vi "Protected Write (0D U8).vi"(8 "error in (no error)":errorcluster, 9 "offset (0)":u64 format="%d bytes", 10 "value in":u8, 11 "Pointer in":refnum<class "Pointer.lvclass">) -> (0 "error out":errorcluster, 1 "offset out":u64 format="%d bytes", 2 "value out":u8, 3 "Pointer out":refnum<class "Pointer.lvclass">)   [LabVIEW 2017, in "Memory Manager.lvlib" / "Pointer.lvclass"]
doc: "Writes the provided <b>value</b> to the address specified by <b>pointer + offset</b>.\n\n<b>Note:</b> This VI is <b>safe</b>.\n\nSafe means that this function evaluates the size parameter of <b>pointer</b> to ensure that is inbounds of allocated memory before peforming a memory read/write. Reading/writing more data to a pointer than it has allocated can corrupt or crash LabVIEW."
uses:
  Pointer.lvclass
  Write/Write (0D U8).vi
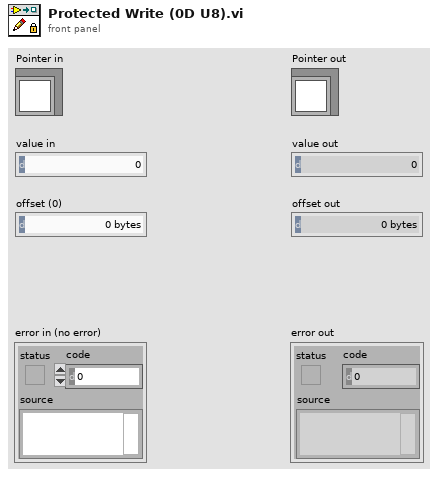
[diagram p1: front panel]
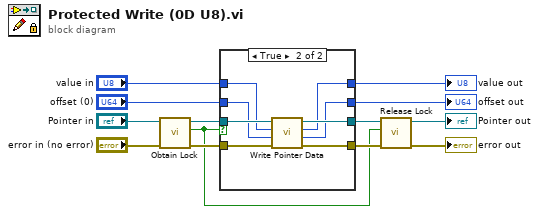
[diagram p0: block diagram]
diagram:
  n1 = call-dynamic "Obtain Lock.vi"("error in (no error)"="error in (no error)", "Pointer in"="Pointer in") -> ("error out"=w11:errorcluster, "lock status"=w9:bool, "Pointer out"=w12:refnum<class "Pointer.lvclass">)  [unwired: 6 in, 1 out]
  n2 = case shown="True" w9 {
    tunnel: [w17 w25] -> w13
    tunnel: [w14 w24] -> w3
    tunnel: [w15 w23] -> w4
    tunnel: w12 -> [w17 w22]
    tunnel: w11 -> [w16 w21]
    tunnel: "value in" -> [w14 w20]
    tunnel: "offset (0)" -> [w15 w19]
    tunnel: [w16 w18] -> w10
    frame False {
    }
    frame True {
      n3 = call-poly "Write Pointer Data.vi"("error in (no error)"=w21, "offset (0)"=w19, "value"=w20, "Pointer in"=w22) -> ("error out"=w18:errorcluster, "offset out"=w23:u64, "value"=w24:u8, "Pointer out"=w25:refnum<class "Pointer.lvclass">)  [unwired: 4 in]
    }
  }
  "value out" <- w3
  "offset out" <- w4
  n4 = call-dynamic "Release Lock.vi"("error in (no error)"=w10, "new lock status (T)"=w9, "Pointer in"=w13) -> ("error out"=→"error out":errorcluster, "Pointer out"=→"Pointer out":refnum<class "Pointer.lvclass">)  [unwired: 6 in, 1 out]
